vi "PH_ImageCoG_Plotter.allocate or free img space.vi"(0 "i ref in":refnum<vi>, 2 "Allocate?":bool, 5 "error in (no error)":errorcluster) -> (14 "i ref out":refnum<vi>, 19 "error out":errorcluster)   [LabVIEW 2014, in "PH_ImageCoG_Plotter.lvlib"]
doc: "This VI is forseen to be used in constructor or destructor. If Allocate? = true is chosen, memory space for several images is allocated. If false is chosen, it is freed."
uses:
  PH_ImageCoG_Plotter.lvlib
  CSCore/CSSystem/CSSystemLib/CSSystemLib.lvlib
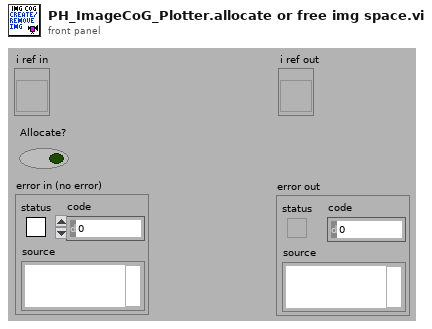
[diagram p1: front panel]
types:
  T1 = typedef "PH_ImageCoG_Plotter.lvlib/PH_ImageCoG_Plotter.i attribute.ctl" = cluster{"GUI Refs":cluster{"Delete":refnum<vi>, "Calibration status":refnum<vi>, "BI subtracted":refnum<vi>, "calc Beam Anal":refnum<vi>, "CoG - x":refnum<vi>, "CoG - y":refnum<vi>, "Type":refnum<vi>, "Center":refnum<vi>, "exp - X":refnum<vi>, "exp - Y":refnum<vi>, "Delta - X":refnum<vi>, "Delta - Y":refnum<vi>, "Available Cams":refnum<vi>, "CoG X":refnum<vi>, "CoG Y":refnum<vi>, "Delta X":refnum<vi>, "Delta Y":refnum<vi>, "Export Data":refnum<vi>, "Calibration data":refnum<vi>}, "Calibration":cluster{"Status":T2, "Calibration data":T3, "Calibration Data File":path}, "Beam Analysis":cluster{"on":bool, "exp - X":i32, "exp - Y":i32, "Type":bool, "Data":cluster{"current time":timestamp, "CoG-x":dbl, "CoG-y":dbl, "Delta-x":dbl, "Delta-y":dbl}[], "Datasets strored":i32, "Dataarray Size":i32}, "Cam instances":string[], "DIM Service Events":T4[], "Images":cluster{"Background":T7, "OP":T7, "GUI":T7}}
  T2 = typedef "PH_StatusHandler.lvlib/PH_StatusHandler.Status.ctl" = i16
  T3 = typedef "PH_ImageCalibrator.lvlib/PH_ImageCalibrator.Calibration Data.ctl" = cluster{"Date":string, "Time":string, "Cam Settings":cluster{"Cam ID":string, "Gain":dbl, "Brightness":dbl, "Shutter":dbl, "Cam Error":bool, "Mode":i32}, "Background Image":cluster{"Image":dbl[][], "Image Error":bool}, "Linear Calibration":cluster{"Calibration Factor":dbl, "not mm or mrad":bool}, "Energy Calibration":cluster{"Calibration Factor":dbl, "no mJ":bool}}
  T4 = typedef "BaseProcess.lvlib/BaseProcess.event definition.ctl" = cluster{"CAEEvtDef":T5, "Data Descriptor":T6}
  T5 = typedef "CAEObj.lvlib/CAEObj.event definition.ctl" = cluster{"URL":string, "enable":bool, "ignoreResID":bool}
  T6 = typedef "BaseProcess.lvlib/BaseProcess.descriptor string definition.ctl" = string
  T7 = typedef "IMAQ Image.ctl" = refnum<image>
  T8 = typedef "Image Type" = u32
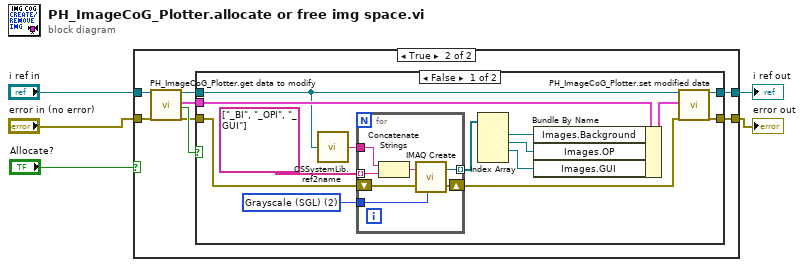
[diagram p0: block diagram]
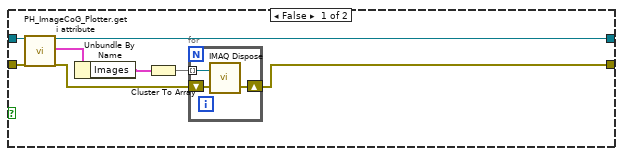
[diagram p2: hidden frame]
diagram:
  n1 = case shown="True" "Allocate?" {
    tunnel: [w8 w23] -> w5
    tunnel: [w10 w22] -> w4
    tunnel: "error in (no error)" -> [w13 w19]
    tunnel: "i ref in" -> [w12 w18]
    frame False {
      n2 = call "PH_ImageCoG_Plotter.get i attribute.vi"("i ref in"=w12, "error in (no error)"=w13) -> ("i ref out"=w10:refnum<vi>, "i attribute"=w11:T1, "error out"=w9:errorcluster)  [unwired: 15 in]
      n3 = Unbundle By Name(w11) -> ("Images"=w7:cluster{"Background":T7, "OP":T7, "GUI":T7})
      n4 = Cluster To Array(cluster=w7) -> (array=w6:T7[])
      n5 = for {
        shift-right: [w15] -> w8
        shift-left: w9 -> [w16]
        tunnel: w6 -> [w14] mode=indexing
        n6 = call "IMAQ Dispose"("Image"=w14, "error in (no error)"=w16) -> ("error out"=w15:errorcluster)  [unwired: 4 in]
      }
    }
    frame True {
      n7 = call "PH_ImageCoG_Plotter.get data to modify.vi"("i ref in"=w18, "error in (no error)"=w19) -> ("i ref out"=w21:refnum<vi>, "i attribute"=w17:T1, "timed out"=w24:bool, "error out"=w20:errorcluster)  [unwired: 14 in]
      n8 = case shown="False" w24 {
        tunnel: w20 -> [w33 w46]
        tunnel: w21 -> [w26 w47]
        tunnel: [w38 w47] -> w22
        tunnel: [w37 w46] -> w23
        tunnel: w17 -> [w36 _]
        frame False {
          w28 = T8 2 items=["Grayscale (U8)", "Grayscale (I16)", "Grayscale (SGL)", "Complex (CSG)", "RGB (U32)", "HSL (U32)", "RGB (U64)"] ("Image Type")
          n9 = call "CSSystemLib.ref2name.vi"("obj refnum"=w26) -> ("name"=w25:string)
          n10 = for {
            shift-right: [w45] -> w34
            shift-left: w33 -> [w44]
            tunnel: [w39] -> w32 mode=indexing
            tunnel: string[] ["_BI", "_OPI", "_GUI"] -> [w41] mode=indexing
            tunnel: w28 -> [w43]
            tunnel: w25 -> [w42]
            n11 = Concatenate Strings(w42, w41) -> (w40:string)
            n12 = call "IMAQ Create"("Image Name"=w40, "Image Type"=w43, "error in (no error)"=w44) -> ("New Image"=w39:T7, "error out"=w45:errorcluster)  [unwired: 2 in]
          }
          n13 = Index Array(array=w32) -> (element #1=w30:T7, element #2=w29:T7, element #3=w27:T7)  [unwired: 4 in, 1 out]
          n14 = Bundle By Name(cluster=w36, "Images.Background"=w30, "Images.OP"=w29, "Images.GUI"=w27) -> (w35:T1)
          n15 = call "PH_ImageCoG_Plotter.set modified data.vi"("i ref in"=w26, "i attribute"=w35, "error in (no error)"=w34) -> ("i ref out"=w38:refnum<vi>, "error out"=w37:errorcluster)  [unwired: 15 in]
        }
        frame True {
        }
      }
    }
  }
  "error out" <- w5
  "i ref out" <- w4
